vi "UV-VIS RAWDATA clean_up.vi"(6 "BG":i32, 7 "All?":bool=TRUE, 8 "error in (no error)":errorcluster, 9 "# of scan":i32, 10 "channel":i32[][](array[numeric]), 11 "UV-VIS in":refnum<class "CCD_camera.lvclass">) -> (0 "error out":errorcluster, 1 "channel seq":cluster{"BG":i32[], "Ie":i32[], "I0":i32[]}[](array[cluster]), 3 "UV-VIS out":refnum<class "CCD_camera.lvclass">)   [LabVIEW 2018, in "CCD_camera.lvclass"]
uses:
  CCD_camera.lvclass
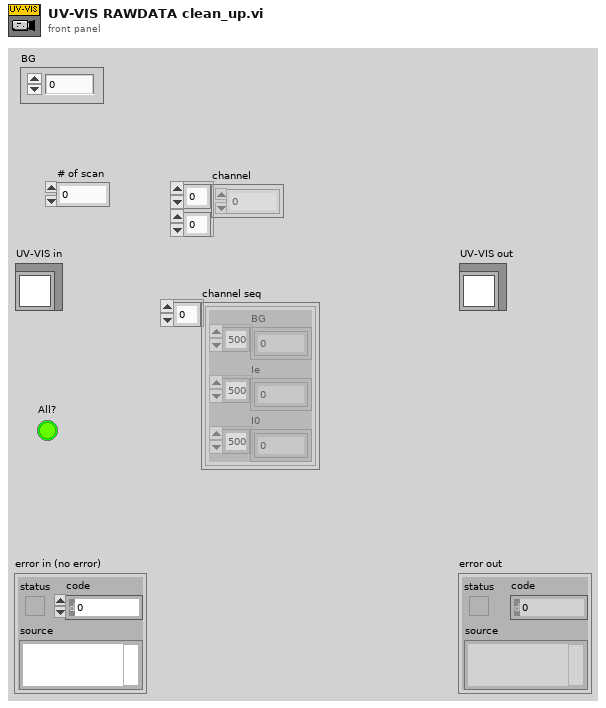
[diagram p1: front panel]
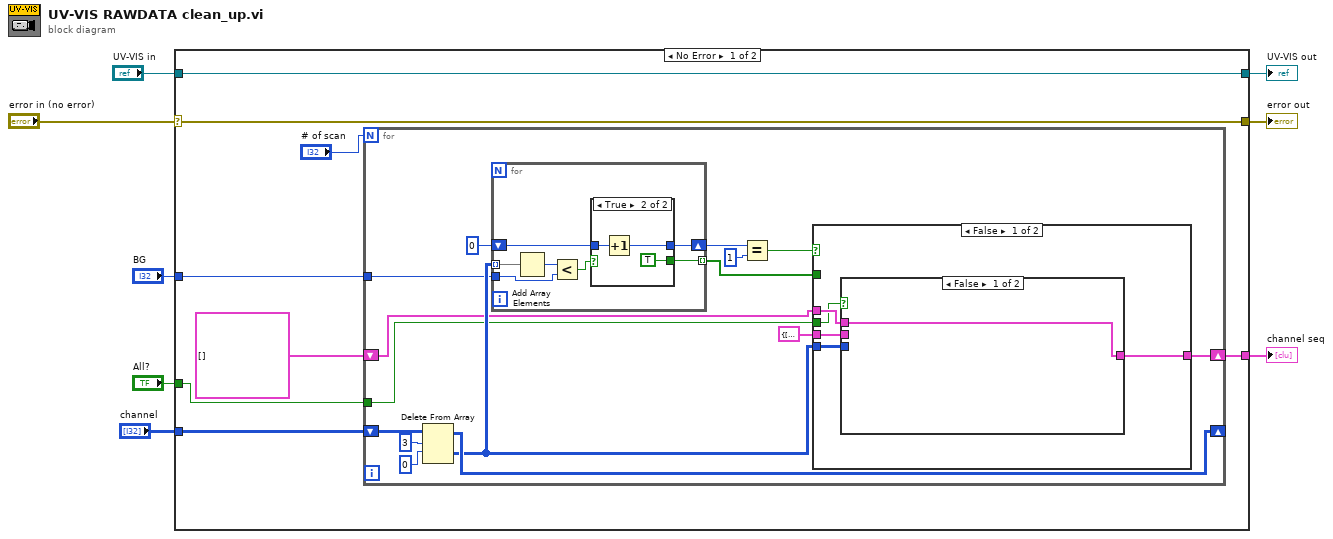
[diagram p0: block diagram]
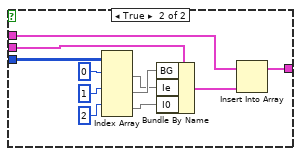
[diagram p2: hidden frame]
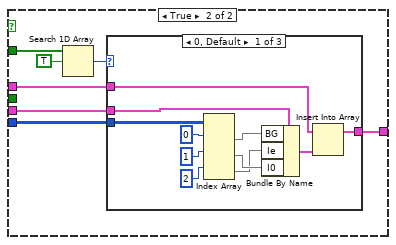
[diagram p3: hidden frame]
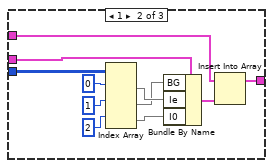
[diagram p4: hidden frame]
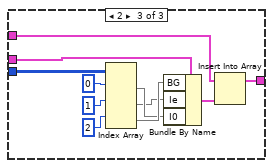
[diagram p5: hidden frame]
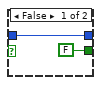
[diagram p6: hidden frame]
diagram:
  n1 = case shown="No Error" "error in (no error)" {
    selector: "error in (no error)" -> [w15 w102]
    tunnel: [w15 w102] -> w5
    tunnel: [w16 w101] -> w7
    tunnel: "UV-VIS in" -> [w16 w101]
    tunnel: "All?" -> [w12 _]
    tunnel: "BG" -> [w11 _]
    tunnel: "channel" -> [w10 _]
    tunnel: [w9 _] -> w1
    frame No Error {
      n2 = for {
        N: "# of scan" -> [_]
        shift-right: [w29] -> _
        shift-left: w10 -> [w19]
        shift-right: [w21] -> w9
        shift-left: cluster{"BG":u16[], "Ie":u16[], "I0":u16[]}[] [] -> [w22]
        tunnel: w12 -> [w18]
        tunnel: w11 -> [w17]
        n3 = Delete From Array(array=w19, length=3 ("longueur"), index (row)=0 ("indice (ligne)")) -> (deleted portion=w23:i32[][], array with subset deleted=w29:i32[][])  [unwired: 1 in]
        n4 = for {
          tunnel: w23 -> [w95] mode=indexing
          tunnel: [w92] -> w24 mode=indexing
          shift-right: [w90] -> w27
          shift-left: 0 -> [w91]
          tunnel: w17 -> [w89]
          n5 = Add Array Elements(numeric array=w95) -> (sum=w94:i32)
          n6 = Less?(x=w94, y=w89) -> (x < y?=w93:bool)
          n7 = case shown="True" w93 {
            tunnel: [FALSE TRUE] -> w92
            tunnel: w91 -> [w96 w99]
            tunnel: [w96 w98] -> w90
            frame False {
            }
            frame True {
              n8 = Increment(x=w99) -> (x+1=w98:i32)
            }
          }
        }
        n9 = Equal?(x=w27, y=1) -> (x = y?=w25:bool)
        n10 = case shown="False" w25 {
          tunnel: w24 -> [_ w55]
          tunnel: w23 -> [w34 w52]
          tunnel: w22 -> [w36 w51]
          tunnel: [w35 w50] -> w21
          tunnel: cluster{"BG":u16[], "Ie":u16[], "I0":u16[]} {"BG"=[], "Ie"=[], "I0"=[]} ("input cluster") -> [w33 w49]
          tunnel: w18 -> [w32 _]
          frame False {
            n11 = case shown="False" w32 {
              tunnel: w36 -> [w37 w41]
              tunnel: [w37 w40] -> w35
              tunnel: w34 -> [_ w39]
              tunnel: w33 -> [_ w38]
              frame False {
              }
              frame True {
                n12 = Index Array(array=w39, index (row) #1=0 ("index (row)"), index (row) #2=1 ("index (row)"), index (row) #3=2 ("index (row)")) -> (element #1=w45:i32[], element #2=w47:i32[], element #3=w46:i32[])  [unwired: 3 in]
                n13 = Bundle By Name(cluster=w38, "BG"=w47, "Ie"=w45, "I0"=w46) -> (w48:cluster{"BG":u16[], "Ie":u16[], "I0":u16[]})
                n14 = Insert Into Array(array=w41, new element=w48) -> (w40:cluster{"BG":u16[], "Ie":u16[], "I0":u16[]}[])  [unwired: 1 in]
              }
            }
          }
          frame True {
            n15 = Search 1D Array(1D array=w55, element=TRUE) -> (index of element=w53:i32)  [unwired: 1 in]
            n16 = case shown="0, Default" w53 {
              tunnel: w52 -> [w63 w74 w85]
              tunnel: w51 -> [w58 w69 w81]
              tunnel: [w57 w68 w79] -> w50
              tunnel: w49 -> [w56 w67 w78]
              frame 0, Default {
                n17 = Index Array(array=w63, index (row) #1=0 ("index (row)"), index (row) #2=1 ("index (row)"), index (row) #3=2 ("index (row)")) -> (element #1=w62:i32[], element #2=w61:i32[], element #3=w60:i32[])  [unwired: 3 in]
                n18 = Bundle By Name(cluster=w56, "BG"=w62, "Ie"=w60, "I0"=w61) -> (w59:cluster{"BG":u16[], "Ie":u16[], "I0":u16[]})
                n19 = Insert Into Array(array=w58, new element=w59) -> (w57:cluster{"BG":u16[], "Ie":u16[], "I0":u16[]}[])  [unwired: 1 in]
              }
              frame 1 {
                n20 = Index Array(array=w74, index (row) #1=0 ("index (row)"), index (row) #2=1 ("index (row)"), index (row) #3=2 ("index (row)")) -> (element #1=w73:i32[], element #2=w71:i32[], element #3=w72:i32[])  [unwired: 3 in]
                n21 = Bundle By Name(cluster=w67, "BG"=w71, "Ie"=w73, "I0"=w72) -> (w70:cluster{"BG":u16[], "Ie":u16[], "I0":u16[]})
                n22 = Insert Into Array(array=w69, new element=w70) -> (w68:cluster{"BG":u16[], "Ie":u16[], "I0":u16[]}[])  [unwired: 1 in]
              }
              frame 2 {
                n23 = Index Array(array=w85, index (row) #1=0 ("index (row)"), index (row) #2=1 ("index (row)"), index (row) #3=2 ("index (row)")) -> (element #1=w83:i32[], element #2=w82:i32[], element #3=w84:i32[])  [unwired: 3 in]
                n24 = Bundle By Name(cluster=w78, "BG"=w84, "Ie"=w82, "I0"=w83) -> (w80:cluster{"BG":u16[], "Ie":u16[], "I0":u16[]})
                n25 = Insert Into Array(array=w81, new element=w80) -> (w79:cluster{"BG":u16[], "Ie":u16[], "I0":u16[]}[])  [unwired: 1 in]
              }
            }
          }
        }
      }
    }
    frame Error {
    }
  }
  "UV-VIS out" <- w7
  "error out" <- w5
  "channel seq" <- w1
